vi "Ultrasonic.vi"(1 "Enum":T1) -> (0 "Distance":dbl)   [LabVIEW 2014]
uses:
  <vilib>/Rock Robotics/SystemInterfaces/AI/FPGA_AIChannel.ctl
  <vilib>/Rock Robotics/WPI/Ultrasonic/WPI_SonarSRF04DigitalOpen.vi
  <vilib>/Rock Robotics/WPI/Ultrasonic/WPI_SonarSRF04DigitalGetRange.vi
  <vilib>/Rock Robotics/WPI/Ultrasonic/WPI_SonarSRF04DigitalClose.vi
  TypeDefs/SRE Enum.ctl
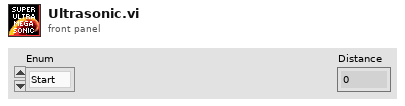
[diagram p1: front panel]
types:
  T1 = typedef "SRE Enum.ctl" = enum16{"Start", "Run", "End"}
  T2 = typedef "FPGA_AIChannel.ctl" = enum8{"AI 0", "AI 1", "AI 2", "AI 3", "AI MXP 0", "AI MXP 1", "AI MXP 2", "AI MXP 3", "Invalid"}
  T3 = typedef "WPI_UltrasonicDeviceRef.ctl" = cluster{"DevStatus":errorcluster, "Ping Digital Controller":T4, "Echo Digital Controller":T4, "Ping Channel":T5, "Echo Channel":T5, "CntIndex":T6}
  T4 = typedef "FPGA_TypedefDigitalModule.ctl" = enum16{"Controller 1"}
  T5 = typedef "FPGA_DIOChannel.ctl" = enum8{"DIO 0", "DIO 1", "DIO 2", "DIO 3", "DIO 4", "DIO 5", "DIO 6", "DIO 7", "DIO 8", "DIO 9", "DIO MXP 0", "DIO MXP 1", "DIO MXP 2", "DIO MXP 3", "DIO MXP 4", "DIO MXP 5", "DIO MXP 6", "DIO MXP 7", "DIO MXP 8", "DIO MXP 9", "DIO MXP 10", "DIO MXP 11", "DIO MXP 12", "DIO MXP 13", "DIO MXP 14", "DIO MXP 15", "Invalid"}
  T6 = typedef "FPGA_CounterCtrSystemIndex.ctl" = enum8{"Ctr 0", "Ctr 1", "Ctr 2", "Ctr 3", "Ctr 4", "Ctr 5", "Ctr 6", "Ctr 7", "Invalid"}
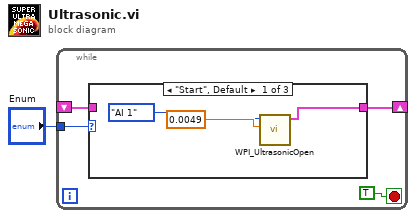
[diagram p0: block diagram]
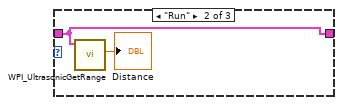
[diagram p2: hidden frame]
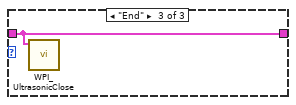
[diagram p3: hidden frame]
diagram:
  n1 = while {
    tunnel: "Enum" -> [w5]
    shift-right: [w2] -> _
    shift-left: _ -> [w3]
    stop <- TRUE stop-if-true
    n2 = case shown="\"Start\", Default" w5 {
      tunnel: w3 -> [_ w9 w11]
      tunnel: [w6 w9 w11] -> w2
      frame "Start", Default {
        n3 = call-poly <vilib>:"WPI_UltrasonicOpen.vi"("Echo Controller"=0.0049 ("Scaling factor (V/in)"), "Ping DIO Channel"=FPGA_AIChannel."AI 1" ("Analog Channel")) -> ("UltrasonicDevRef"=w6:T3)  [unwired: 8 in, 1 out]
      }
      frame "Run" {
        n4 = call-poly <vilib>:"WPI_UltrasonicGetRange.vi"("UltrasonicDevRef"=w9) -> ("Distance"=→"Distance":dbl)  [unwired: 8 in, 2 out]
      }
      frame "End" {
        n5 = call-poly <vilib>:"WPI_UltrasonicClose.vi"("UltrasonicDevRef"=w11) -> ()  [unwired: 10 in, 1 out]
      }
    }
  }
